vi "BasicFlow.vi"(0 "VI Reference In":refnum<vi>, 1 "Label (VI Title)":string="Default", 11 "error in (no error)":errorcluster) -> (4 "VI Reference Out":refnum<vi>, 15 "error out":errorcluster)   [LabVIEW 2016, in "DronaTest.lvlib"]
uses:
  DronaTest.lvlib
  APIs/Stimulus/ValueSignal/ValueSignalByPathString.vi
  apis/Assert/AssertControlValue/Equal.vi
  <vilib>/addons/_JKI Toolkits/Caraya/classes/Assert/Assert Not Error.vi
  <vilib>/addons/_JKI Toolkits/Caraya/classes/Test/Test.lvclass
  Drona.lvlib
  <vilib>/addons/_JKI Toolkits/Caraya/classes/Assert/Assert.lvclass
  apis/Assert/AssertControlValue/AssertControlValue.lvlib
  apis/Stimulus/ValueSignal/ValueSignal.lvlib
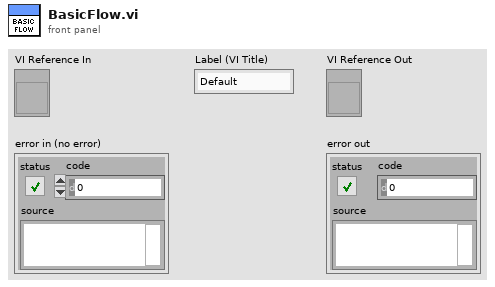
[diagram p1: front panel]
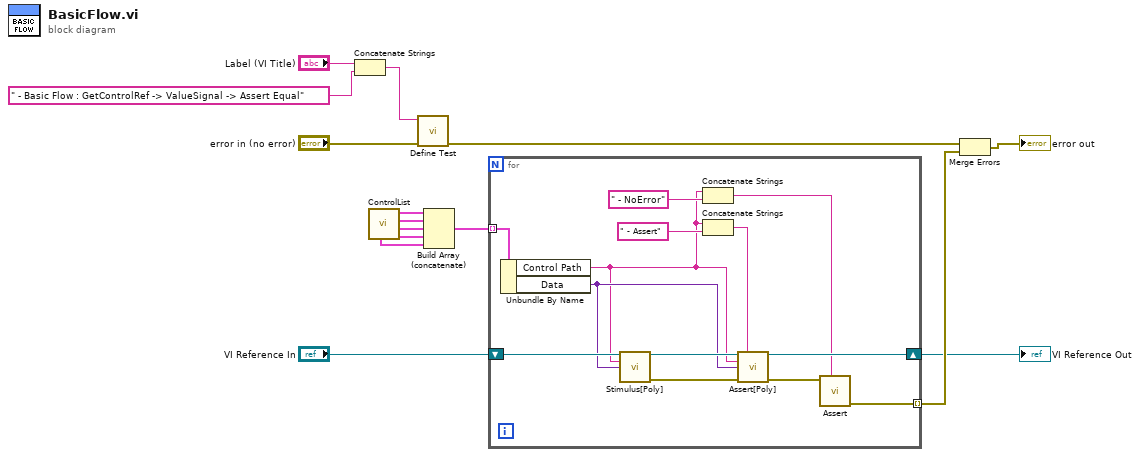
[diagram p0: block diagram]
diagram:
  n1 = Concatenate Strings("Label (VI Title)", " - Basic Flow : GetControlRef -> ValueSignal -> Assert Equal" ("Label (VI Title)")) -> (w6:string)
  n2 = call "ControlList.vi"() -> ("Tab Control"=w2:cluster{"Control Path":string, "Data":variant}[], "BigCluster"=w3:cluster{"Control Path":string, "Data":variant}[], "Cluster"=w4:cluster{"Control Path":string, "Data":variant}[], "Basic"=w10:cluster{"Control Path":string, "Data":variant}[], "BasicArray"=w1:cluster{"Control Path":string, "Data":variant}[])  [unwired: 6 in, 1 out]
  n3 = call <vilib>:"Define Test.vi"("error in (no error)"="error in (no error)", "Label (VI Title)"=w6) -> ("error out"=w9:errorcluster)  [unwired: 9 in]
  n4 = Build Array (concatenate)(w10, w4, w3, w2, w1) -> (w5:cluster{"Control Path":string, "Data":variant}[])
  n5 = for {
    shift-right: [w28] -> w12
    shift-left: "VI Reference In" -> [w24]
    tunnel: [w16] -> w15 mode=indexing
    tunnel: w5 -> [w25] mode=indexing
    n6 = Unbundle By Name(w25) -> ("Control Path"=w19:string, "Data"=w23:variant)
    n7 = call-poly "Stimulus[Poly].vi"("VI Reference In"=w24, "Control Path"=w19, "Value (Signaling)"=w23) -> ("VI Reference Out"=w26:refnum<vi>, "error out"=w27:errorcluster)  [unwired: 11 in]
    n8 = Concatenate Strings(w19, " - NoError" ("string")) -> (w17:string)
    n9 = Concatenate Strings(w19, " - Assert" ("string")) -> (w21:string)
    n10 = call-poly "Assert[Poly].vi"("VI Reference In"=w26, "Label"=w21, "Control Path"=w19, "Control Value"=w23, "Error In"=w27) -> ("VI Reference Out"=w28:refnum<vi>, "Error Out"=w18:errorcluster)  [unwired: 9 in]
    n11 = call-poly <vilib>:"Assert.vi"("Label"=w17, "Not Error?"=w18) -> ("error out"=w16:errorcluster)  [unwired: 9 in]
  }
  "VI Reference Out" <- w12
  n12 = Merge Errors(w9, w15) -> (→"error out":errorcluster)
